vi "Get VMS Data.vi"(10 "VMS Data Type":string, 11 "Clust Refnum":refnum<vi>) -> (3 "Array":dbl[][](array[numeric]))   [LabVIEW 2016, in "M1M3SupportEUI_Views.lvlib"]
uses:
  M1M3SupportEUI_Views.lvlib
  SALLV_vms/DataTypes/M1M3.ctl
  SALLV_vms/SALLV_vms.lvlib
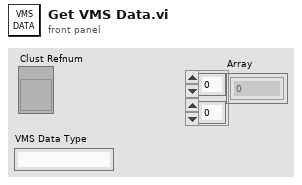
[diagram p1: front panel]
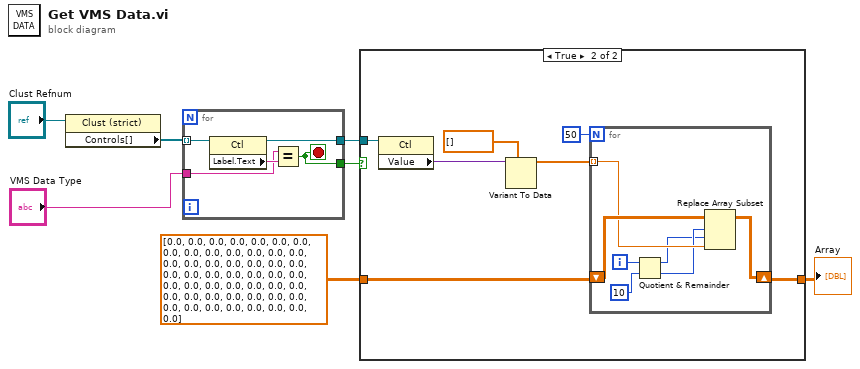
[diagram p0: block diagram]
diagram:
  n1 = property on="Property Node" class="Clust (strict)"(reference="Clust Refnum") -> ("Controls[]"=w6:refnum<vi>[])  [unwired: 1 in, 2 out]
  n2 = for {
    tunnel: w6 -> [w12] mode=indexing
    tunnel: [w11] -> w5
    tunnel: "VMS Data Type" -> [w9]
    tunnel: [w8] -> w4
    stop <- w8 stop-if-true
    n3 = property on="Property Node" class="Ctl"(reference=w12) -> (reference out=w11:refnum<vi>, "Label.Text"=w10:string)  [unwired: 1 in, 1 out]
    n4 = Equal?(x=w9, y=w10) -> (x = y?=w8:bool)
  }
  n5 = case shown="True" w4 {
    tunnel: w5 -> [_ w20]
    tunnel: [w13 w14] -> w1
    tunnel: sgl[][] [[0.0, 0.0, 0.0, 0.0, 0.0, 0.0, 0.0, 0.0, 0.0, 0.0], [0.0, 0.0, 0.0, 0.0, 0.0, 0.0, 0.0, 0.0, 0.0, 0.0], [0.0, 0.0, 0.0, 0.0, 0.0, 0.0, 0.0, 0.0, 0.0, 0.0], [0.0, 0.0, 0.0, 0.0, 0.0, 0.0, 0.0, 0.0, 0.0, 0.0], [0.0, 0.0, 0.0, 0.0, 0.0, 0.0, 0.0, 0.0, 0.0, 0.0]] -> [w13 w17]
    frame False {
    }
    frame True {
      n6 = property on="Property Node" class="Ctl"(reference=w20) -> ("Value"=w19:variant)  [unwired: 1 in, 2 out]
      n7 = Variant To Data(type=sgl[] [], Variant=w19) -> (data=w16:sgl[])  [unwired: 1 in, 1 out]
      n8 = for {
        N: 50 -> [_]
        tunnel: w16 -> [w25] mode=indexing
        shift-right: [w26] -> w14
        shift-left: w17 -> [w27]
        i -> [w24]
        n9 = Quotient & Remainder(x=w24, y=10) -> (x-y*floor(x/y)=w21:i32, floor(x/y)=w22:i32)
        n10 = Replace Array Subset(array=w27, new element=w25, index (row)=w22, index (col)=w21) -> (w26:sgl[][])
      }
    }
  }
  "Array" <- w1
